vi "RunSAS.vi"(8 "error in":errorcluster, 11 "AirSAS Controls":T1={"Receive Duration"=0.0, "I/O"={"DAQmx Device"="Dev1", "AO Range"=0.0, "AI Range"=0.0, "DAQ Group Delay"=0.0, "Fs"=0.0}, "Hardware"={"Centerpos"=[], "TXpos"=[], "RX1pos"=[], "RX2pos"=[], "Angle"=0.0, "Height"=0.0}, "Waveform"={"LFM Parameters"={"Duration"=1.0, "Fstart (Hz)"=1000.0, "Fstop (Hz)"=10000.0, "Out. Amplitude (Vpk)"=1.0, "Window %"=10.0}, "Transmit Waveform"={"t0"=timestamp(0 s since 1904-01-01), "dt"=1.0, "Y"=[]}}, "LINX Resource"={"IO"=enum."Remote", "Interface"=enum."Serial", "LINX Device Config"={"Interface"=enum."Serial", "COM Port"="COM13", "TCP Configuration"={"IP Address"="", "Port"=0}, "Device Family"=1, "Device ID"=1, "Device Name"="myRIO-1900", "TCP Ref"=refnum, "Channels"={"DI"=[0, 1, 2, 3, 4, 5, 6, 7, 8, 9, 10, 11, 12, 13, 14, 15, 16, 17, 18, 19, 20, 21, 22, 23, 24, 25, 26, 27, 28, 29, 30, 31, 32, 33, 34, 35, 36, 37, 38, 39, 40, 41, 42, 43, 44, 45, 46], "DO"=[0, 1, 2, 3, 4, 5, 6, 7, 8, 9, 10, 11, 12, 13, 14, 15, 16, 17, 18, 19, 20, 21, 22, 23, 24, 25, 26, 27, 28, 29, 30, 31, 32, 33, 34, 35, 36, 37, 38, 39, 40, 41, 42, 43, 44, 45, 46], "AI"=[0, 1, 2, 3, 4, 5, 6, 7, 8, 9, 10, 11], "AO"=[], "PWM"=[3, 5, 6, 9, 10], "QE"=[], "UART"=[0, 1], "I2C 2"=[0], "SPI"=[0], "CAN"=[], "Servo"=[], "AI Ref (V)"=0.0, "AI Resolution (Bits)"=0, "AO Ref (V)"=0.0, "AO Resolution (Bits)"=0}}}, "Port"=3000.0} {"Waveform"."LFM Parameters"."Window %" format="%.2g"; "Waveform"."LFM Parameters"."Out. Amplitude (Vpk)" format="%0.2f"; "Waveform"."LFM Parameters"."Fstop (Hz)" format="%^.3e"; "Waveform"."LFM Parameters"."Fstart (Hz)" format="%^.3e"; "Waveform"."LFM Parameters"."Duration" format="%.3f"}) -> (0 "error out":errorcluster, 3 "AirSAS Controls 2":T1={"Receive Duration"=0.0, "I/O"={"DAQmx Device"="Dev1", "AO Range"=0.0, "AI Range"=0.0, "DAQ Group Delay"=0.0, "Fs"=0.0}, "Hardware"={"Centerpos"=[], "TXpos"=[], "RX1pos"=[], "RX2pos"=[], "Angle"=0.0, "Height"=0.0}, "Waveform"={"LFM Parameters"={"Duration"=1.0, "Fstart (Hz)"=1000.0, "Fstop (Hz)"=10000.0, "Out. Amplitude (Vpk)"=1.0, "Window %"=10.0}, "Transmit Waveform"={"t0"=timestamp(0 s since 1904-01-01), "dt"=1.0, "Y"=[]}}, "LINX Resource"={"IO"=enum."Remote", "Interface"=enum."Serial", "LINX Device Config"={"Interface"=enum."Serial", "COM Port"="COM13", "TCP Configuration"={"IP Address"="", "Port"=0}, "Device Family"=1, "Device ID"=1, "Device Name"="myRIO-1900", "TCP Ref"=refnum, "Channels"={"DI"=[0, 1, 2, 3, 4, 5, 6, 7, 8, 9, 10, 11, 12, 13, 14, 15, 16, 17, 18, 19, 20, 21, 22, 23, 24, 25, 26, 27, 28, 29, 30, 31, 32, 33, 34, 35, 36, 37, 38, 39, 40, 41, 42, 43, 44, 45, 46], "DO"=[0, 1, 2, 3, 4, 5, 6, 7, 8, 9, 10, 11, 12, 13, 14, 15, 16, 17, 18, 19, 20, 21, 22, 23, 24, 25, 26, 27, 28, 29, 30, 31, 32, 33, 34, 35, 36, 37, 38, 39, 40, 41, 42, 43, 44, 45, 46], "AI"=[0, 1, 2, 3, 4, 5, 6, 7, 8, 9, 10, 11], "AO"=[], "PWM"=[3, 5, 6, 9, 10], "QE"=[], "UART"=[0, 1], "I2C 2"=[0], "SPI"=[0], "CAN"=[], "Servo"=[], "AI Ref (V)"=0.0, "AI Resolution (Bits)"=0, "AO Ref (V)"=0.0, "AO Resolution (Bits)"=0}}}, "Port"=3000.0} {"Waveform"."LFM Parameters"."Window %" format="%.2g"; "Waveform"."LFM Parameters"."Out. Amplitude (Vpk)" format="%0.2f"; "Waveform"."LFM Parameters"."Fstop (Hz)" format="%^.3e"; "Waveform"."LFM Parameters"."Fstart (Hz)" format="%^.3e"; "Waveform"."LFM Parameters"."Duration" format="%.3f"})   [LabVIEW 2021]
uses:
  controls/Air SAS Controls.ctl
  <vilib>/MakerHub/LINX/Private/Type Defs/LINX Ref.ctl
  <vilib>/MakerHub/LINX/Private/Type Defs/Platform.ctl
  <vilib>/MakerHub/LINX/Private/Type Defs/Interface.ctl
  <vilib>/MakerHub/LINX/Private/Device/Type Defs/LINX Device Config.ctl
  <vilib>/MakerHub/LINX/Private/Device/Type Defs/TCP Config.ctl
  <vilib>/MakerHub/LINX/Private/Device/Type Defs/Channels.ctl
  <vilib>/Analysis/4window.llb/Cosine Tapered Window (DBL).vi
  <vilib>/Waveform/WDTOps.llb/WDT Number of Waveform Samples DBL.vi
  <vilib>/Analysis/NI_AALBase.lvlib
  <vilib>/Analysis/NI_AALPro.lvlib
  <vilib>/MakerHub/LINX/LMH-LINX.lvlib
  <vilib>/MakerHub/LINX/Private/Device/Device.lvlib
panel:
  in  "Folder Path":path=path "C:/Users/jqn5303/Desktop/testfiles"
  out "Gauge":cluster{dbl, dbl, dbl}(knob)={0.0, -178.0803549193409, -96.36742372843878} scale format="%#_g°"
  out "Slide":cluster{dbl, dbl, dbl}(slide)={0.0, 227.2365805168986, 42.94234592445328} scale=0.0..900.0
  in  "Averages":dbl=1.0 min=1.0 step=1.0
  in  "Receive Duration":dbl=0.01
  out "Acquired Data":waveform(dbl)(graph)
  in  "Start Acquisition":bool
  in  "Motion Control":T8={"SAS Geometry"=enum."Circular", "Angular Step"=1.0, "Vertical Step"=0.0, "Vertical Min"=0.0, "Vertical Max"=0.0, "Angular Start"=1.0, "Angular Stop"=20.0}
  in  "stop":bool
  in  "Generate LFM":bool
  out "Transmit Waveform":waveform(dbl)(graph)
  in  "LFM Parameters":T9={"Fs (Hz)"=100000.0, "Sweep Length (s)"=0.001, "Fstart (Hz)"=10000.0, "Fstop (Hz)"=10000.0, "Out. Amplitude (Vpk)"=1.0, "Window %"=10.0} {"Window %" format="%.2g"; "Out. Amplitude (Vpk)" format="%0.2f"; "Fstop (Hz)" format="%^.3e"; "Fstart (Hz)" format="%^.3e"; "Sweep Length (s)" format="%.3f"; "Fs (Hz)" min=1000.0 max=2000000.0 format="%^.0e"}
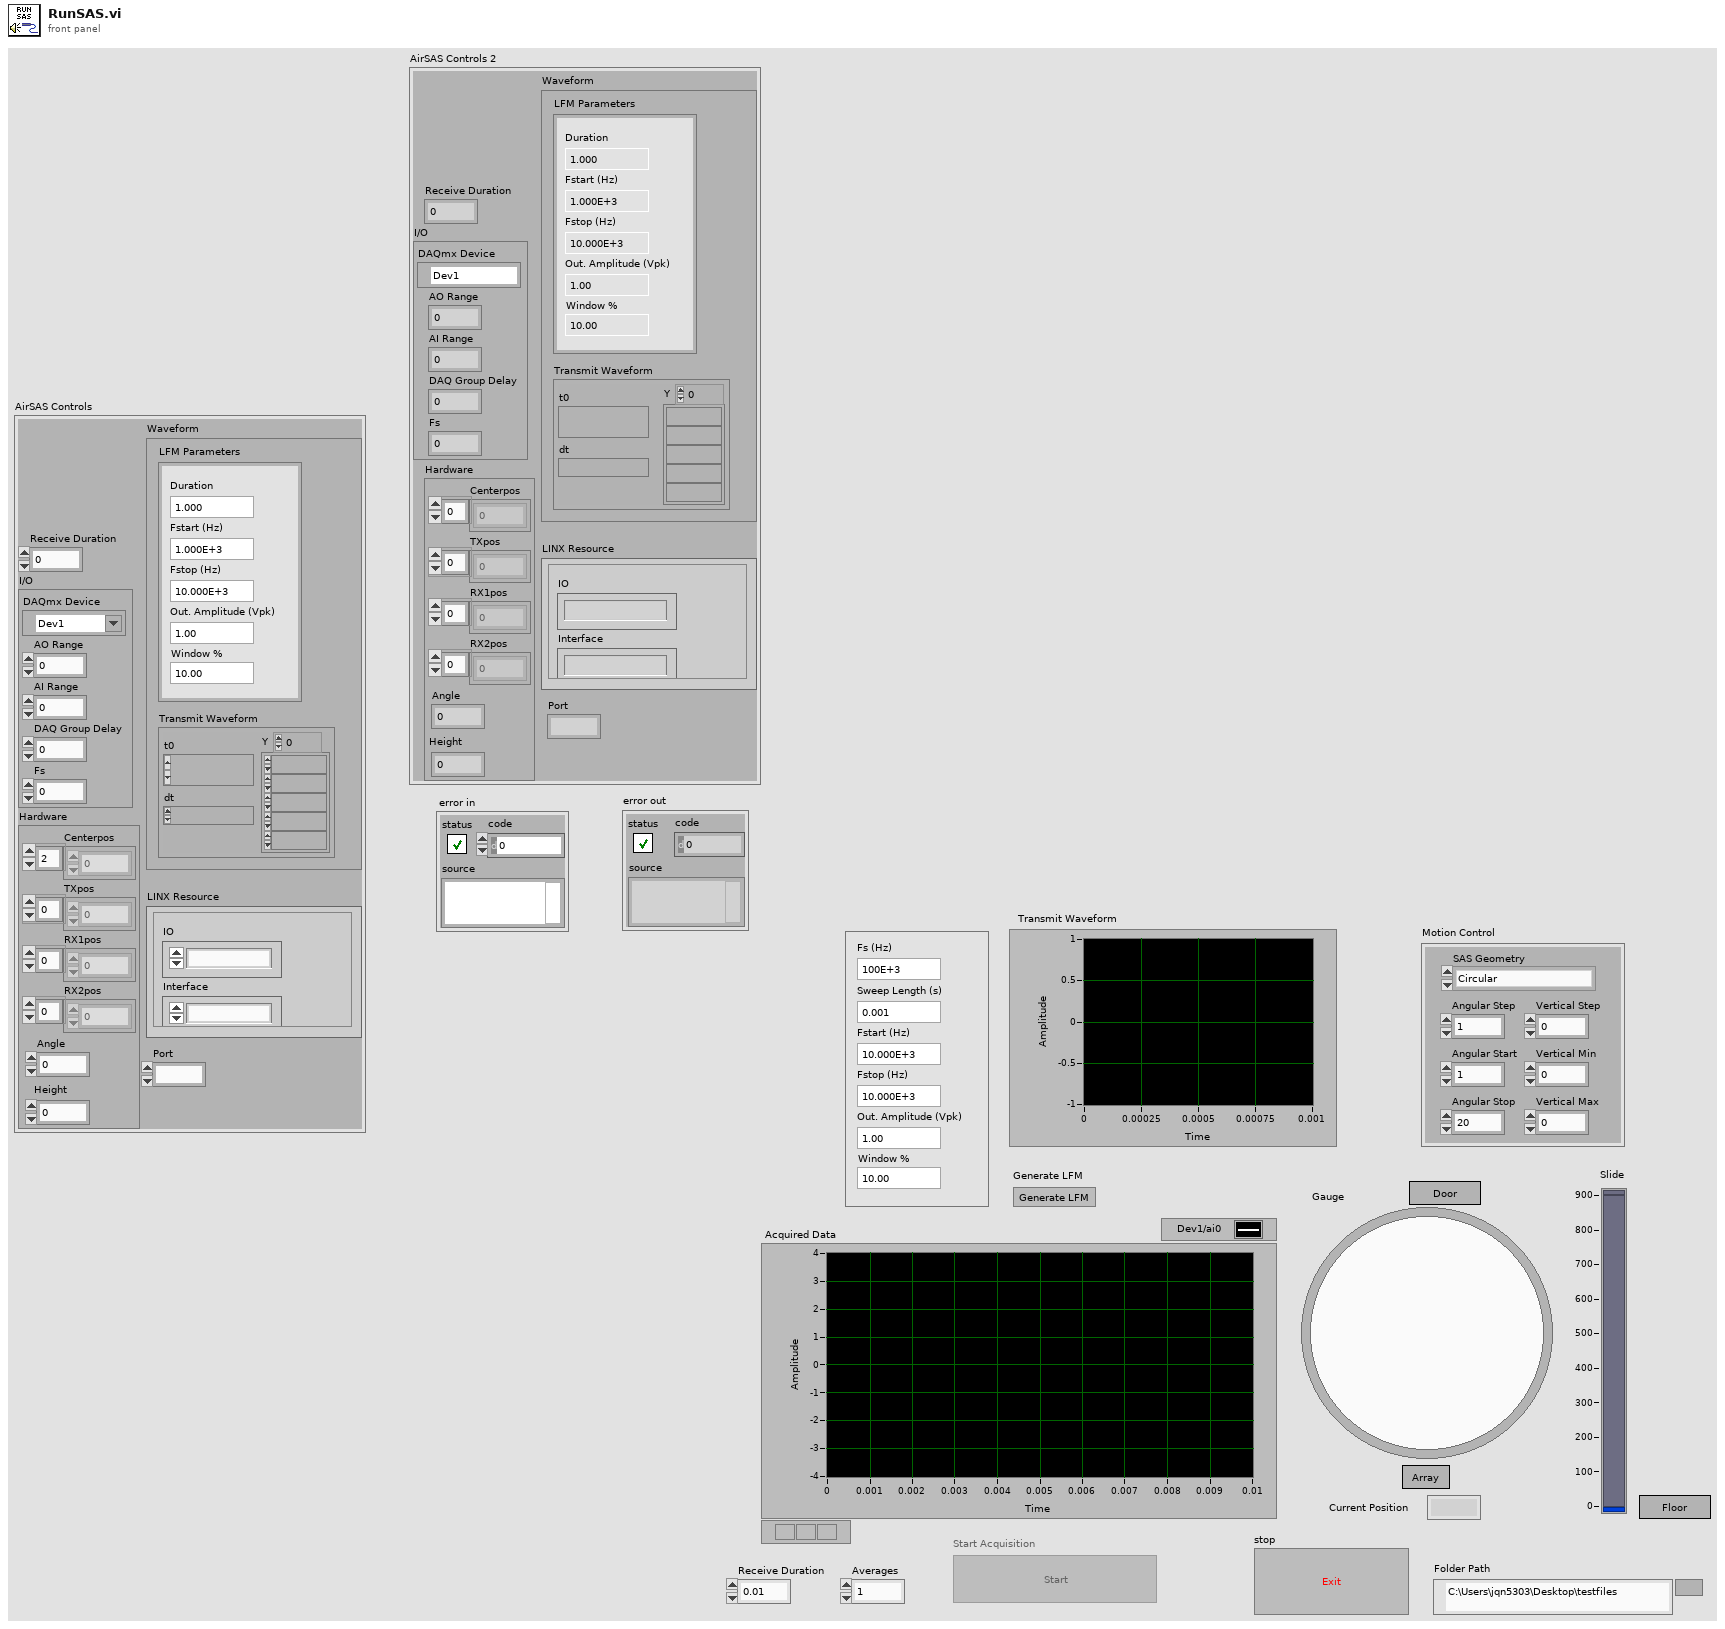
[diagram p1: front panel]
types:
  T1 = typedef "Air SAS Controls.ctl" = cluster{"Receive Duration":dbl, "I/O":cluster{"DAQmx Device":tag, "AO Range":dbl, "AI Range":dbl, "DAQ Group Delay":dbl, "Fs":dbl}, "Hardware":cluster{"Centerpos":dbl[], "TXpos":dbl[], "RX1pos":dbl[], "RX2pos":dbl[], "Angle":dbl, "Height":dbl}, "Waveform":cluster{"LFM Parameters":cluster{"Duration":dbl, "Fstart (Hz)":dbl, "Fstop (Hz)":dbl, "Out. Amplitude (Vpk)":dbl, "Window %":dbl}, "Transmit Waveform":waveform(dbl)}, "LINX Resource":T2, "Port":dbl}
  T2 = typedef "LMH-LINX.lvlib/LINX Ref.ctl" = cluster{"IO":T3, "Interface":T4, "LINX Device Config":T5}
  T3 = typedef "LMH-LINX.lvlib/Platform.ctl" = enum16{"Remote", "Local"}
  T4 = typedef "LMH-LINX.lvlib/Interface.ctl" = enum16{"Serial", "TCP"}
  T5 = typedef "LMH-LINX.lvlib/Device.lvlib/LINX Device Config.ctl" = cluster{"Interface":T4, "COM Port":refnum<visa-resource-name>, "TCP Configuration":T6, "Device Family":u8, "Device ID":u8, "Device Name":string, "TCP Ref":refnum<k5>, "Channels":T7}
  T6 = typedef "LMH-LINX.lvlib/Device.lvlib/TCP Config.ctl" = cluster{"IP Address":string, "Port":u16}
  T7 = typedef "LMH-LINX.lvlib/Channels.ctl" = cluster{"DI":u8[], "DO":u8[], "AI":u8[], "AO":u8[], "PWM":u8[], "QE":u8[], "UART":u8[], "I2C 2":u8[], "SPI":u8[], "CAN":u8[], "Servo":u8[], "AI Ref (V)":dbl, "AI Resolution (Bits)":u8, "AO Ref (V)":dbl, "AO Resolution (Bits)":u8}
  T8 = cluster{"SAS Geometry":enum16{"Circular", "Cylindrical", "Spiral"}, "Angular Step":dbl, "Vertical Step":dbl, "Vertical Min":dbl, "Vertical Max":dbl, "Angular Start":dbl, "Angular Stop":dbl}
  T9 = cluster{"Fs (Hz)":dbl, "Sweep Length (s)":dbl, "Fstart (Hz)":dbl, "Fstop (Hz)":dbl, "Out. Amplitude (Vpk)":dbl, "Window %":dbl}
  T10 = enum8{"Enabled", "Disabled", "Disabled and Grayed Out"}
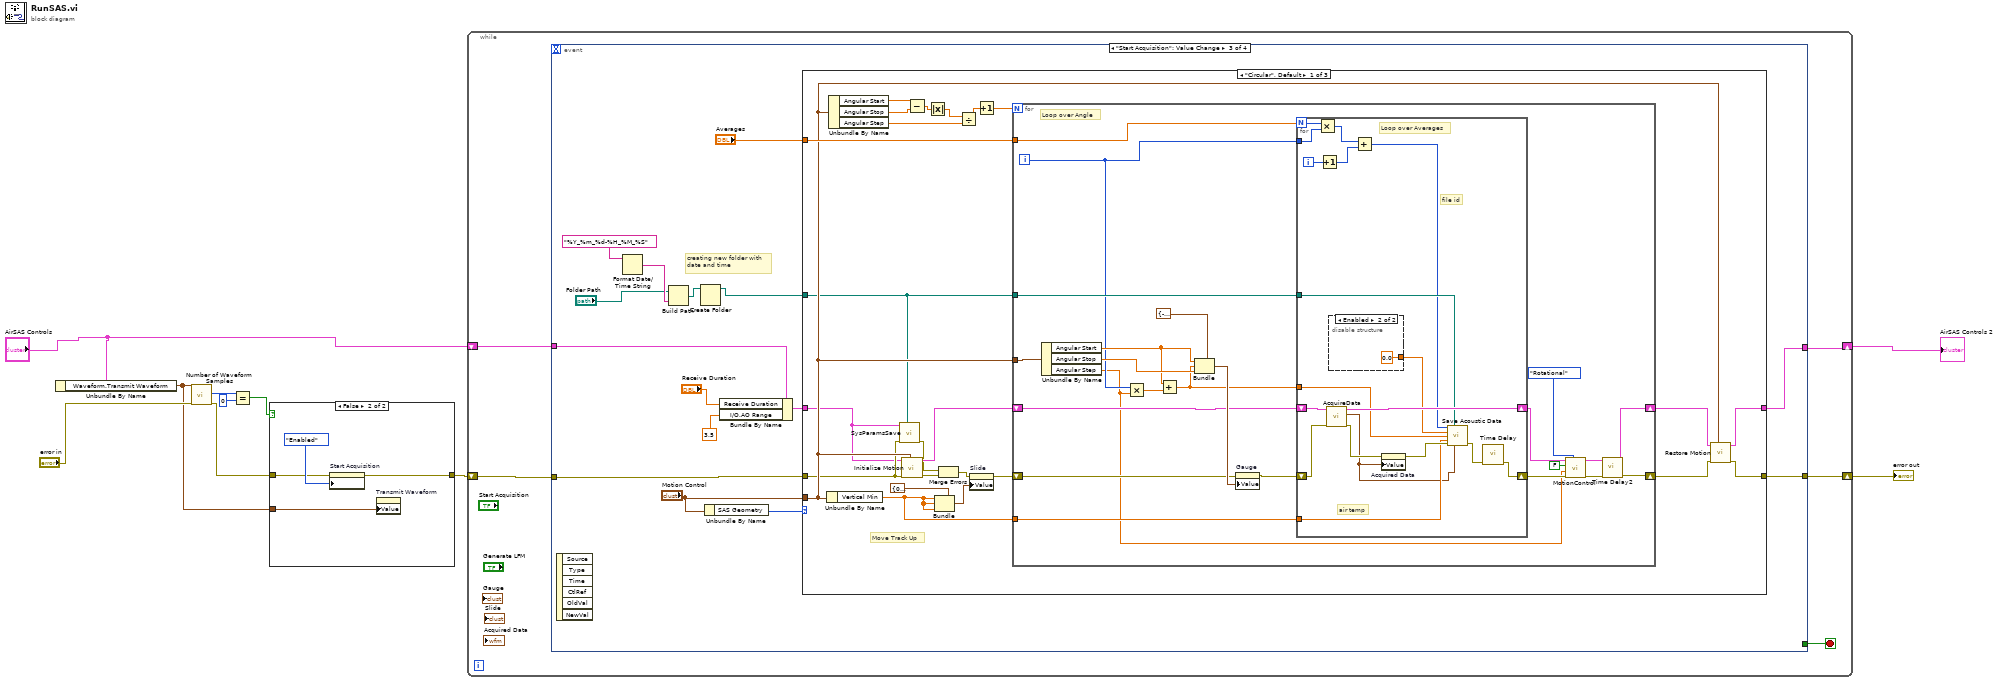
[diagram p0: block diagram]
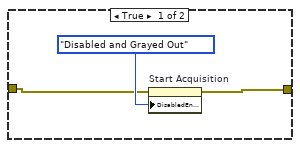
[diagram p2: hidden frame]
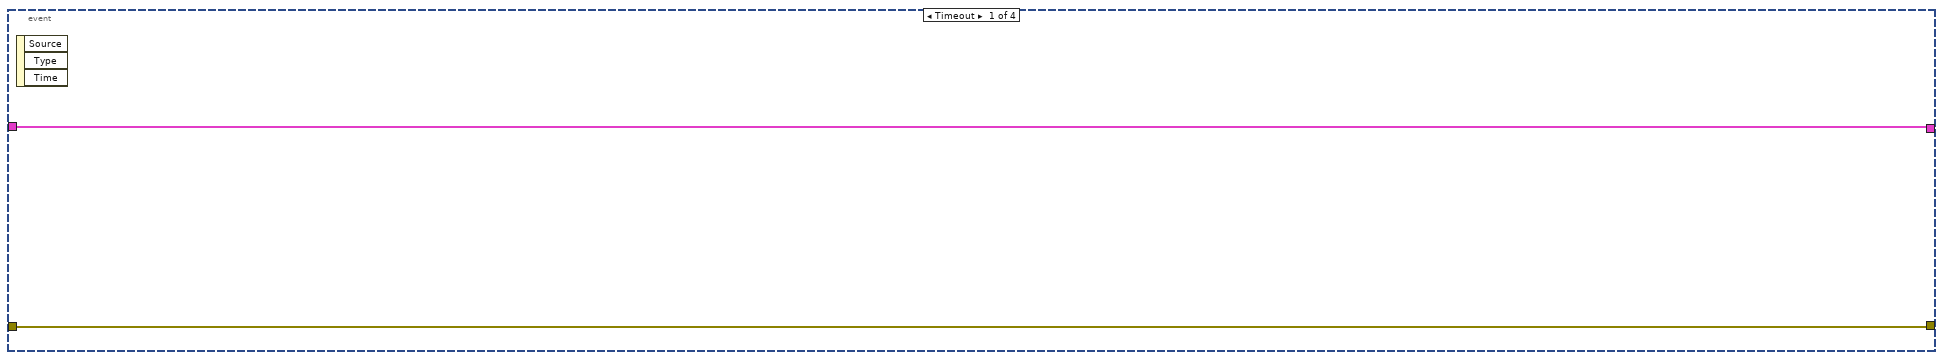
[diagram p3: hidden frame]
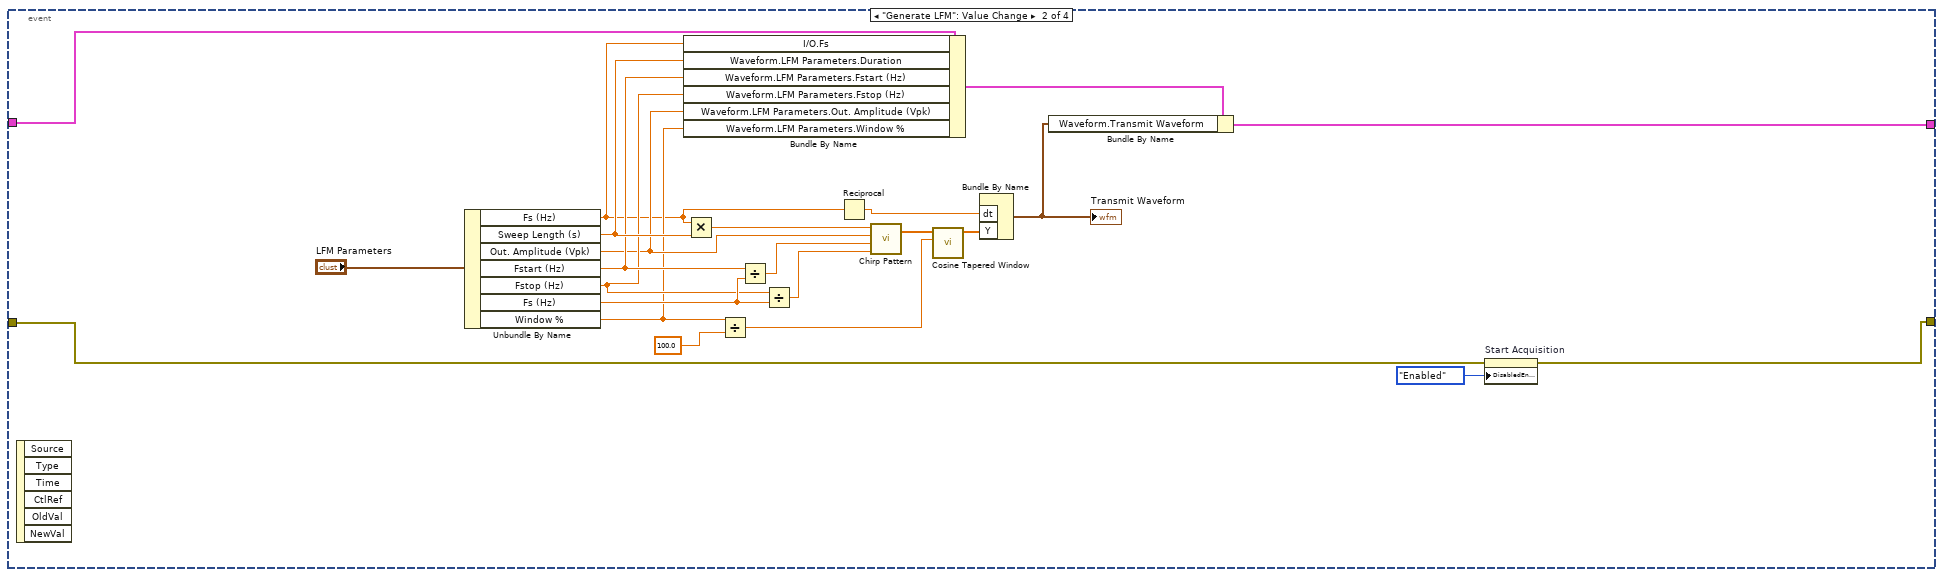
[diagram p4: hidden frame]
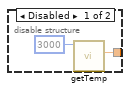
[diagram p5: hidden frame]
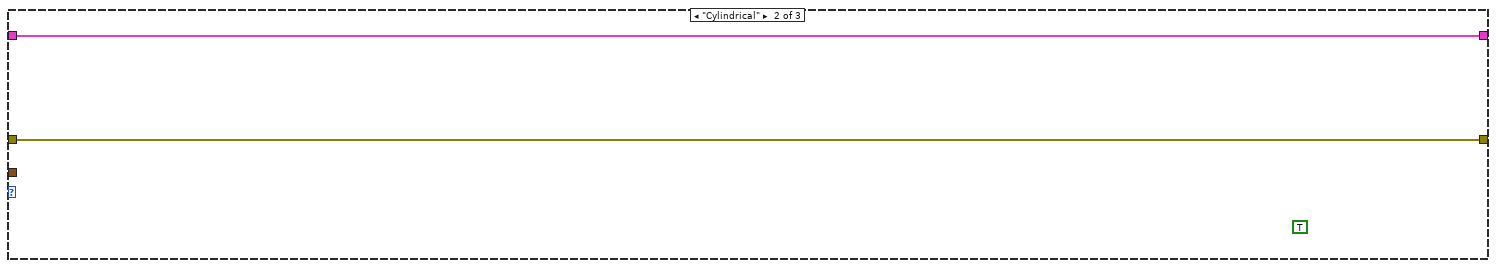
[diagram p6: hidden frame]
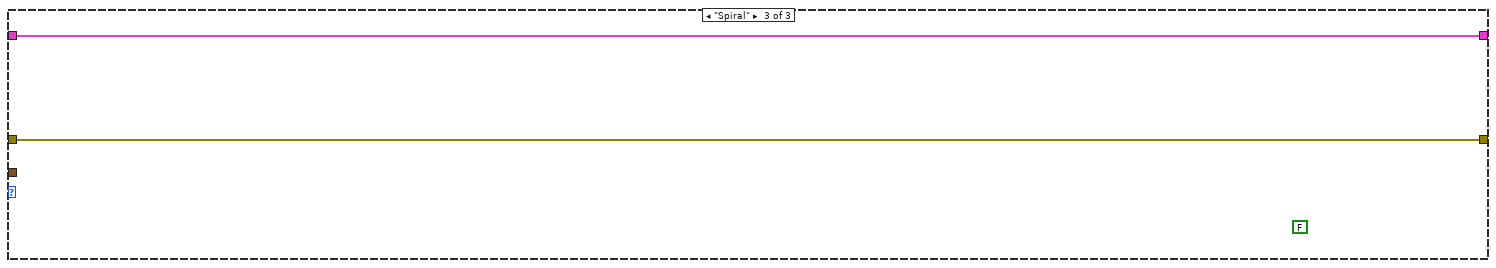
[diagram p7: hidden frame]
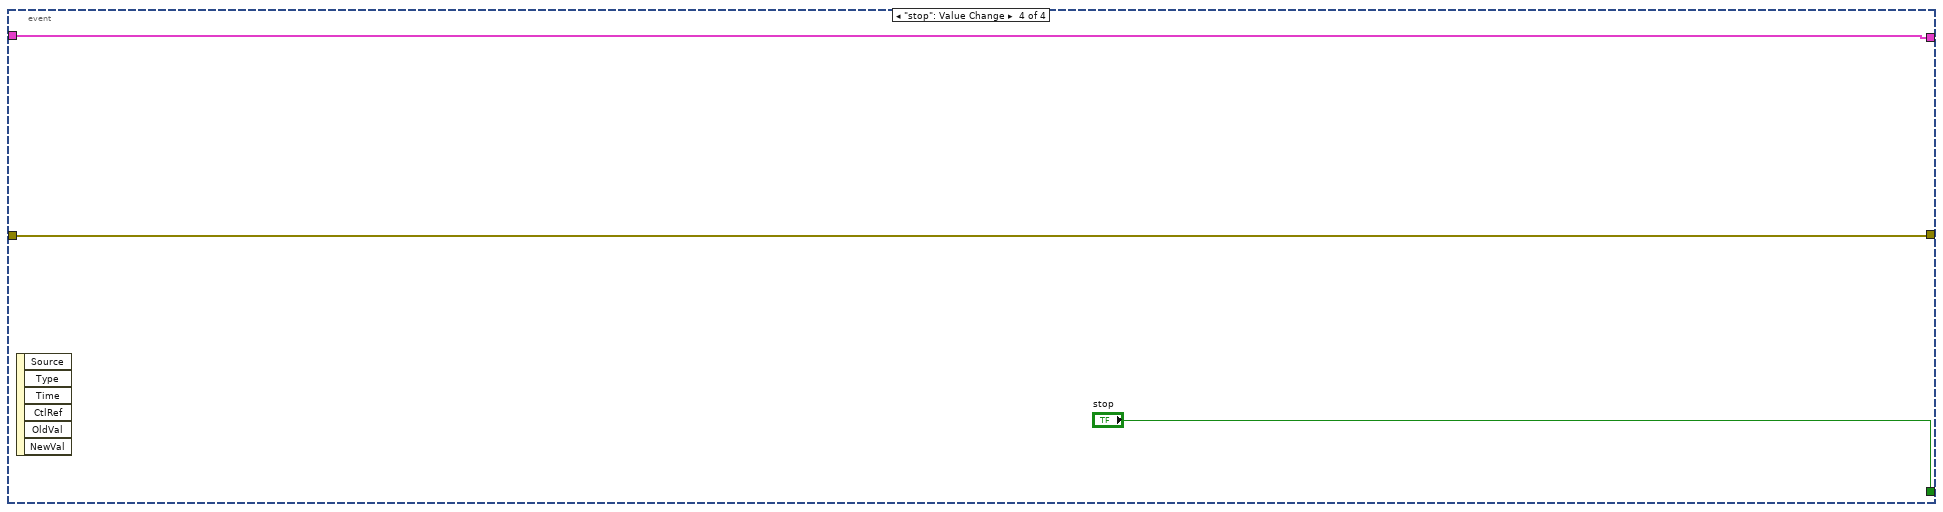
[diagram p8: hidden frame]
diagram:
  n1 = Unbundle By Name("AirSAS Controls") -> ("Waveform.Transmit Waveform"=w3:waveform(dbl))
  n2 = call-poly <vilib>:"Number of Waveform Samples.vi"("error in (no error)"="error in", "waveform in"=w3) -> ("error out"=w4:errorcluster, "number of samples"=w9:i32)  [unwired: 7 in, 1 out]
  n3 = Equal?(x=w9, y=0) -> (x = y?=w7:bool)
  n4 = case shown="False" w7 {
    tunnel: [w11 w15] -> w5
    tunnel: w4 -> [w12 w14]
    tunnel: w3 -> [_ w16]
    frame True {
      n5 = property on="Start Acquisition" class="Bool"(error in=w12, "DisabledEnum"=T10."Disabled and Grayed Out" ("Disabled")) -> (error out=w11:errorcluster)  [unwired: 1 in, 1 out]
    }
    frame False {
      n6 = property on="Start Acquisition" class="Bool"(error in=w14, "DisabledEnum"=T10."Enabled" ("Disabled")) -> (error out=w15:errorcluster)  [unwired: 1 in, 1 out]
      n7 = property on="Transmit Waveform" class="WFGraph (strict)"("Value"=w16) -> ()  [unwired: 2 in, 2 out]
    }
  }
  n8 = while {
    shift-right: [w21] -> w1
    shift-left: "AirSAS Controls" -> [w22]
    shift-right: [w18] -> w10
    shift-left: w5 -> [w19]
    stop <- w20 stop-if-true
    n9 = event shown="[2] \"Start Acquisition\": Value Change" {
      selector: _ -> [_ _ _ _]
      dyn-events: _ -> [_ _ _ _]
      timeout: _ -> [_ _ _ _]
      tunnel: w22 -> [w24 w37 w61 w135]
      tunnel: [w24 w29 w62 w135] -> w21
      tunnel: [_ _ _ "stop"] -> w20
      tunnel: w19 -> [w23 w26 w54 w134]
      tunnel: [w23 w25 w53 w134] -> w18
      event Timeout {
        n10 = event-data() -> ()  [unwired: 1 in, 3 out]
      }
      event "Generate LFM": Value Change {
        n11 = event-data() -> ()  [unwired: 1 in, 6 out]
        n12 = Unbundle By Name("LFM Parameters") -> ("Fs (Hz)"=w28:dbl, "Sweep Length (s)"=w36:dbl, "Out. Amplitude (Vpk)"=w33:dbl, "Fstart (Hz)"=w35:dbl, "Fstop (Hz)"=w34:dbl, "Fs (Hz)"=w45:dbl, "Window %"=w32:dbl)
        n13 = Bundle By Name(cluster=w37, "I/O.Fs"=w28, "Waveform.LFM Parameters.Duration"=w36, "Waveform.LFM Parameters.Fstart (Hz)"=w35, "Waveform.LFM Parameters.Fstop (Hz)"=w34, "Waveform.LFM Parameters.Out. Amplitude (Vpk)"=w33, "Waveform.LFM Parameters.Window %"=w32) -> (w31:T1)
        n14 = Multiply(x=w28, y=w36) -> (x*y=w47:dbl)
        n15 = Divide(x=w32, y=100.0) -> (x/y=w40:dbl)
        n16 = Divide(x=w35, y=w45) -> (x/y=w46:dbl)
        n17 = Divide(x=w34, y=w45) -> (x/y=w44:dbl)
        n18 = Reciprocal(x=w28) -> (1/x=w41:dbl)
        n19 = call <vilib>:"Chirp Pattern.vi"("f2"=w44, "f1"=w46, "amplitude"=w33, "samples"=w47) -> ("Chirp Pattern"=w43:dbl[])  [unwired: 1 out]
        n20 = call-poly <vilib>:"Cosine Tapered Window.vi"("ratio"=w40, "X"=w43) -> ("Windowed X"=w42:dbl[])  [unwired: 8 in, 1 out]
        n21 = Bundle By Name("dt"=w41, "Y"=w42) -> (w30:waveform(dbl))  [unwired: 1 in]
        "Transmit Waveform" <- w30
        n22 = Bundle By Name(cluster=w31, "Waveform.Transmit Waveform"=w30) -> (w29:T1)
        n23 = property on="Start Acquisition" class="Bool"(error in=w26, "DisabledEnum"=T10."Enabled" ("Disabled")) -> (error out=w25:errorcluster)  [unwired: 1 in, 1 out]
      }
      event "Start Acquisition": Value Change {
        # "creating new folder with\ndate and time"
        n24 = event-data() -> ()  [unwired: 1 in, 6 out]
        n25 = Format Date/Time String(time format string (%c)="%Y_%m_%d-%H_%M_%S") -> (date/time string=w51:string)  [unwired: 2 in]
        n26 = Build Path(base path="Folder Path", name or relative path=w51) -> (appended path=w52:path)
        n27 = Create Folder(path (use dialog)=w52) -> (created path=w48:path)  [unwired: 2 in, 2 out]
        n28 = Unbundle By Name("Motion Control") -> ("SAS Geometry"=w60:enum16{"Circular", "Cylindrical", "Spiral"})
        n29 = Bundle By Name(cluster=w61, "Receive Duration"="Receive Duration", "I/O.AO Range"=3.5) -> (w58:T1)
        n30 = case shown="\"Circular\", Default" w60 {
          tunnel: "Motion Control" -> [w71 _ _]
          tunnel: w58 -> [w68 w131 w133]
          tunnel: [w74 w131 w133] -> w62
          tunnel: w54 -> [w69 w130 w132]
          tunnel: [w72 w130 w132] -> w53
          tunnel: "Averages" -> [w80 _ _]
          tunnel: w48 -> [w70 _ _]
          frame "Circular", Default {
            # "Move Track Up"
            n31 = Unbundle By Name(w71) -> ("Vertical Min"=w76:dbl)
            n32 = Unbundle By Name(w71) -> ("Angular Start"=w64:dbl, "Angular Stop"=w63:dbl, "Angular Step"=w84:dbl)
            n33 = call "SysParamsSave.vi"("Path"=w70, "error in (no error)"=w69, "AirSAS Controls"=w68) -> ("error out"=w65:errorcluster)  [unwired: 8 in]
            n34 = call "Initialize Motion.vi"("Motion Control"=w71, "Error In"=w69, "AirSAS Controls"=w68) -> ("Error Out"=w66:errorcluster, "output cluster"=w77:T1)  [unwired: 7 in]
            n35 = Subtract(x=w64, y=w63) -> (x-y=w86:dbl)
            n36 = Absolute Value(x=w86) -> (abs(x)=w85:dbl)
            n37 = Bundle(cluster=cluster{dbl, dbl, dbl} {0.0, 227.2365805168986, 42.94234592445328} ("Slide 2"), w76, w76, w76) -> (w78:cluster{dbl, dbl, dbl})
            n38 = Merge Errors(w65, w66) -> (w67:errorcluster)
            n39 = Divide(x=w85, y=w84) -> (x/y=w83:dbl)
            n40 = property on="Slide" class="Slide (strict)"(error in=w67, "Value"=w78) -> (error out=w79:errorcluster)  [unwired: 1 in, 1 out]
            n41 = Increment(x=w83) -> (x+1=w81:dbl)
            n42 = for {
              N: w81 -> [_]
              tunnel: w71 -> [w108]
              shift-right: [w97] -> w75
              shift-left: w77 -> [w101]
              shift-right: [w87] -> w73
              shift-left: w79 -> [w104]
              tunnel: w80 -> [w106]
              tunnel: w70 -> [w102]
              tunnel: w76 -> [w100]
              i -> [w90]
              # "Loop over Angle"
              n43 = Unbundle By Name(w108) -> ("Angular Start"=w91:dbl, "Angular Stop"=w94:dbl, "Angular Step"=w89:dbl)
              n44 = Multiply(x=w90, y=w89) -> (x*y=w93:dbl)
              n45 = Add(x=w91, y=w93) -> (x+y=w92:dbl)
              n46 = Bundle(cluster=cluster{dbl, dbl, dbl} {-172.55422153679154, 17.21837893351085, -51.118830131082746} ("Gauge 2"), w91, w92, w94) -> (w105:cluster{dbl, dbl, dbl})
              n47 = property on="Gauge" class="Knob (strict)"(error in=w104, "Value"=w105) -> (error out=w103:errorcluster)  [unwired: 1 in, 1 out]
              n48 = for {
                N: w106 -> [w123]
                tunnel: w90 -> [w122]
                shift-right: [w119] -> w98
                shift-left: w101 -> [w126]
                shift-right: [w110] -> w99
                shift-left: w103 -> [w125]
                tunnel: w102 -> [w116]
                tunnel: w100 -> [w113]
                tunnel: w92 -> [w112]
                i -> [w124]
                # "Loop over Averages"
                # "file id"
                # "air temp"
                n49 = Multiply(x=w123, y=w122) -> (x*y=w121:i32)
                n50 = Increment(x=w124) -> (x+1=w120:i32)
                n51 = call "AcquireData.vi"("error in"=w125, "AirSAS Controls In"=w126) -> ("error out"=w118:errorcluster, "data"=w109:waveform(dbl), "AirSAS Controls Out"=w119:T1)  [unwired: 7 in]
                n52 = disable-structure shown="Enabled" {
                  disable-tunnel: [w128 0.0 ("Air Temperature")] -> w114
                  frame Disabled {
                    n53 = call "getTemp.vi"("port"=u16 3000) -> ("Temp"=w128:dbl)  [unwired: 9 in, 1 out]
                  }
                  frame Enabled {
                  }
                }
                n54 = Add(x=w121, y=w120) -> (x+y=w115:i32)
                n55 = property on="Acquired Data" class="WFGraph (strict)"(error in=w118, "Value"=w109) -> (error out=w117:errorcluster)  [unwired: 1 in, 1 out]
                n56 = call "Save Acoustic Data.vi"("ID"=w115, "base path"=w116, "Air Temperature"=w114, "Angle"=w112, "Height"=w113, "error in (no error)"=w117, "Captured Data"=w109) -> ("error out"=w111:errorcluster)  [unwired: 8 in]
                n57 = call "Time Delay"("error in (no error)"=w111) -> ("error out"=w110:errorcluster)  [unwired: 10 in]
              }
              n58 = call "MotionControl.vi"("Motion Type"=enum16{"Linear", "Rotational"}."Rotational", "Error In"=w99, "Distance"=w89, "Direction"=FALSE, "AirSAS Controls"=w98) -> ("Error Out"=w88:errorcluster, "output cluster"=w97:T1)  [unwired: 5 in]
              n59 = call "Time Delay2"("error in (no error)"=w88) -> ("error out"=w87:errorcluster)  [unwired: 10 in]
            }
            n60 = call "Restore Motion.vi"("Motion Control"=w71, "Error In"=w73, "AirSAS Controls"=w75) -> ("Error Out"=w72:errorcluster, "output cluster"=w74:T1)  [unwired: 7 in]
          }
          frame "Cylindrical" {
            (unwired) TRUE
          }
          frame "Spiral" {
            (unwired) FALSE
          }
        }
      }
      event "stop": Value Change {
        n61 = event-data() -> ()  [unwired: 1 in, 6 out]
      }
    }
  }
  "error out" <- w10
  "AirSAS Controls 2" <- w1
